vi "Get Library Names in Active Project.vi"(8 "error in (no error)":errorcluster, 11 "project ref":refnum<vi>) -> (0 "error out":errorcluster, 3 "library names":string[](array[string]))   [LabVIEW 2021, in "NI Measurement V2 Client Generator Runtime.lvlib"]
uses:
  NI Measurement V2 Client Generator Runtime.lvlib
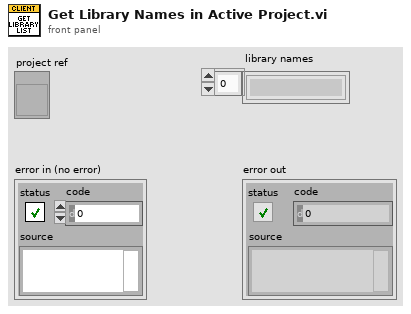
[diagram p1: front panel]
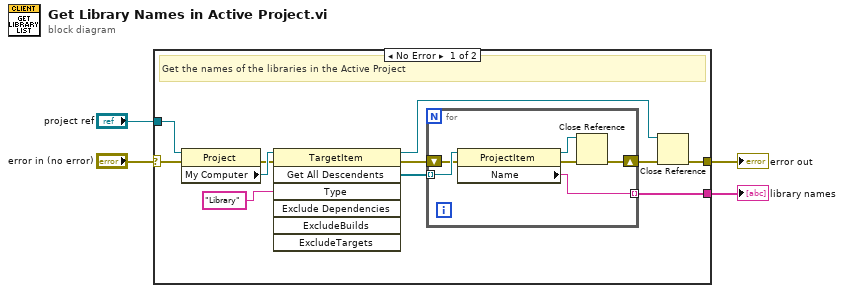
[diagram p0: block diagram]
diagram:
  n1 = case shown="No Error" "error in (no error)" {
    selector: "error in (no error)" -> [w11 w22]
    tunnel: "project ref" -> [w15 _]
    tunnel: [w6 w22] -> w2
    tunnel: [w7 _] -> w1
    frame No Error {
      # "Get the names of the libraries in the Active Project"
      n2 = property class="Project"(reference=w15, error in=w11) -> (error out=w13:errorcluster, "My Computer"=w14:refnum<vi>)  [unwired: 1 out]
      n3 = invoke class="TargetItem" method="Get All Descendents"(reference=w14, error in=w13, "Type"="Library") -> (reference out=w5:refnum<vi>, error out=w9:errorcluster, "All Descendents"=w12:refnum<vi>[])  [unwired: 4 in, 4 out]
      n4 = for {
        tunnel: w12 -> [w21] mode=indexing
        shift-right: [w18] -> w10
        shift-left: w9 -> [w20]
        tunnel: [w16] -> w7 mode=indexing
        n5 = property class="ProjectItem"(reference=w21, error in=w20) -> (reference out=w17:refnum<vi>, error out=w19:errorcluster, "Name"=w16:string)
        n6 = Close Reference(reference=w17, error in (no error)=w19) -> (error out=w18:errorcluster)
      }
      n7 = Close Reference(reference=w5, error in (no error)=w10) -> (error out=w6:errorcluster)
    }
    frame Error {
      # "Pass"
    }
  }
  "error out" <- w2
  "library names" <- w1
